vi "重启设置.vi"() -> ()   [LabVIEW 2016]
uses:
  <vilib>/Utility/miscctls.llb/LVPointTypeDef.ctl
  <vilib>/Utility/config.llb/NI_LVConfig.lvlib
panel:
  in  "取消":bool
  in  "确认":bool
  in  "分":u16=2 max=59 format="%02.0f"
  in  "频次":T1(ring)
  in  "时":u16=2 max=23 format="%02.0f"
  # "请选择要重启的时间点"
  # "频次："
  # "时间："
  # "："
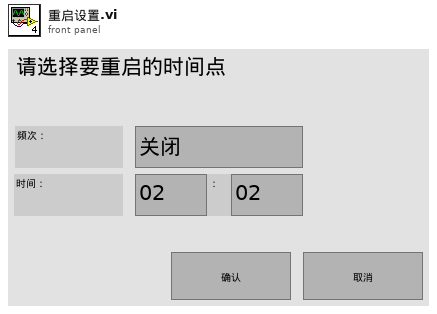
[diagram p1: front panel]
types:
  T1 = enum16{"关闭", "每天", "星期一", "星期二", "星期三", "星期四", "星期五", "星期六", "星期日"}
  T2 = typedef "LVPointTypeDef.ctl" = cluster{"Horizontal":i16, "Vertical":i16}
  T3 = cluster{"频次":enum16{"关闭", "每天", "星期一", "星期二", "星期三", "星期四", "星期五", "星期六", "星期日"}, "时":u16, "分":u16}
  T4 = typedef "NI_LVConfig.lvlib/Config Data RefNum.ctl" = refnum<k1>
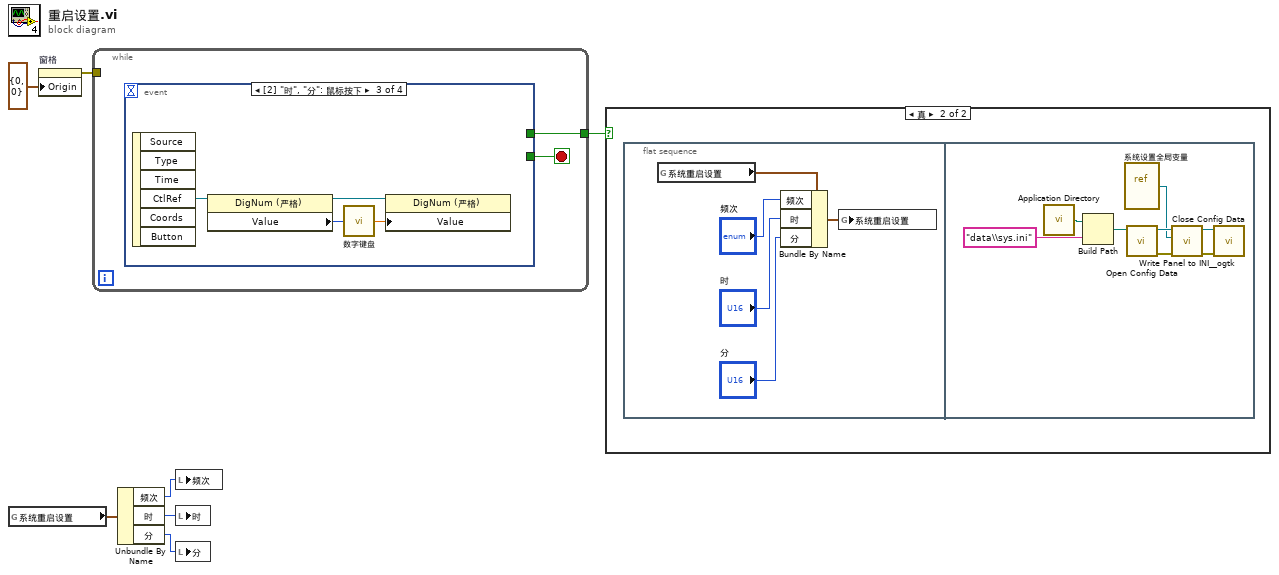
[diagram p0: block diagram]
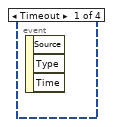
[diagram p3: hidden frame]
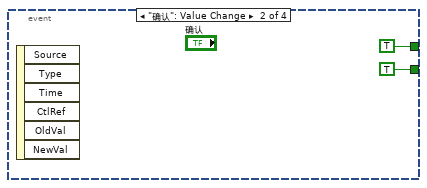
[diagram p4: hidden frame]
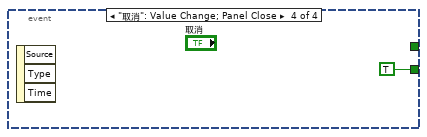
[diagram p5: hidden frame]
diagram:
  n1 = global read "系统设置全局变量.vi" "系统重启设置"() -> (w4:T3)
  n2 = property on="窗格" class="Pane"("Origin"=T2 {"Horizontal"=0, "Vertical"=0} ("原点")) -> (error out=w5:errorcluster)  [unwired: 2 in, 1 out]
  n3 = while {
    tunnel: [w8] -> w7
    tunnel: w5 -> [_]
    stop <- w9 stop-if-true
    n4 = event shown="[2] \"时\", \"分\": 鼠标按下" {
      selector: _ -> [_ _ _ _]
      dyn-events: _ -> [_ _ _ _]
      timeout: _ -> [_ _ _ _]
      tunnel: [_ TRUE _ TRUE] -> w9
      tunnel: [_ TRUE _ _] -> w8
      event Timeout {
        n5 = event-data() -> ()  [unwired: 1 in, 3 out]
      }
      event "确认": Value Change {
        n6 = event-data() -> ()  [unwired: 1 in, 6 out]
      }
      event "时", "分": Mouse Down {
        n7 = event-data() -> ("CtlRef"=w15:refnum<vi>)  [unwired: 1 in, 5 out]
        n8 = property class="DigNum (严格)"(reference=w15) -> (reference out=w14:refnum<vi>, "Value"=w13:u16)  [unwired: 1 in, 1 out]
        n9 = call "数字键盘.vi"("OldNumber"=w13) -> ("NewNumber"=w12:sgl)
        n10 = property class="DigNum (严格)"(reference=w14, "Value"=w12) -> ()  [unwired: 1 in, 2 out]
      }
      event "取消": Value Change; Panel Close {
        n11 = event-data() -> ()  [unwired: 1 in, 3 out]
      }
    }
  }
  n12 = Unbundle By Name(w4) -> ("频次"=w3:T1, "时"=w2:u16, "分"=w1:u16)
  n13 = local write "频次"(w3) -> ()
  n14 = local write "时"(w2) -> ()
  n15 = local write "分"(w1) -> ()
  n16 = case shown="真" w7 {
    frame False {
    }
    frame True {
      n17 = flat-sequence {
        frame #0 {
          n18 = global read "系统设置全局变量.vi" "系统重启设置"() -> (w21:T3)
          n19 = Bundle By Name(cluster=w21, "频次"="频次", "时"="时", "分"="分") -> (w20:T3)
          n20 = global write "系统设置全局变量.vi" "系统重启设置"(w20) -> ()
        }
        frame #1 {
          n21 = call <vilib>:"Application Directory.vi"() -> ("Application Directory"=w29:path)
          n22 = Build Path(base path=w29, name or relative path="data\\sys.ini" ("名称或相对路径")) -> (appended path=w27:path)
          n23 = vi-ref "系统设置全局变量.vi"() -> (w25:refnum<vi>)
          n24 = call <vilib>:"Open Config Data.vi"("configuration file path"=w27) -> ("error out"=w23:errorcluster, "refnum"=w26:T4)  [unwired: 8 in, 1 out]
          n25 = call <userlib>:"Write Panel to INI__ogtk.vi"("error in (no error)"=w23, "VI ref"=w25, "refnum"=w26) -> ("error out"=w22:errorcluster, "refnum out"=w24:T4)  [unwired: 7 in]
          n26 = call <vilib>:"Close Config Data.vi"("error in (no error)"=w22, "refnum"=w24) -> ()  [unwired: 8 in, 2 out]
        }
      }
    }
  }
